vi "Heading.vi"(0 "X Array":dbl[](array[numeric]), 1 "Target X":dbl, 2 "Current X":dbl, 3 "Current Y":dbl, 4 "Target Y":dbl, 5 "Y Array":dbl[](array[numeric]), 7 "stop":bool) -> (6 "Current Heading":dbl, 8 "Desired Heading":dbl)   [LabVIEW 2012]
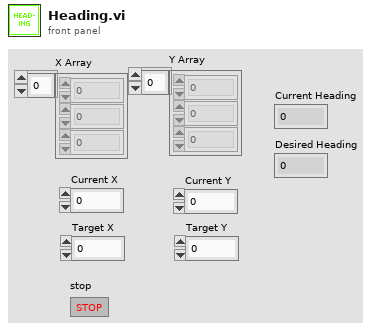
[diagram p1: front panel]
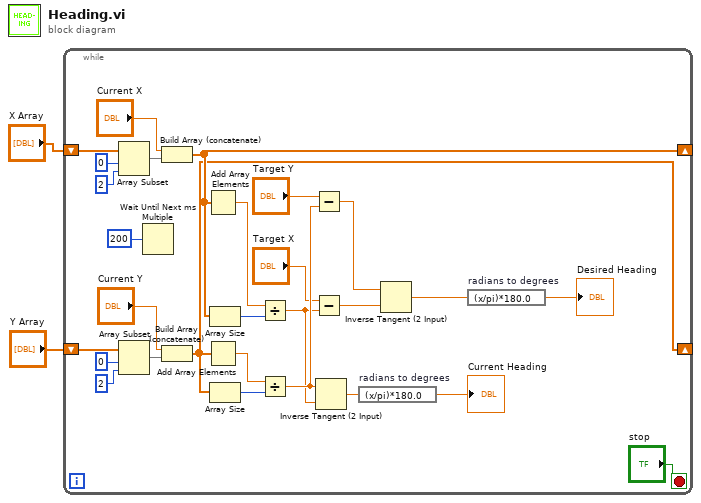
[diagram p0: block diagram]
diagram:
  n1 = while {
    shift-right: [w22] -> _
    shift-left: "X Array" -> [w30]
    shift-right: [w13] -> _
    shift-left: "Y Array" -> [w14]
    stop <- "stop" stop-if-true
    n2 = Array Subset(array=w30, index=0, length=2) -> (w27:dbl[])
    n3 = Array Subset(array=w14, index=0, length=2) -> (w18:dbl[])
    n4 = Wait Until Next ms Multiple(millisecond multiple=200) -> ()  [unwired: 1 out]
    n5 = Build Array (concatenate)("Current X", w27) -> (w22:dbl[])
    n6 = Build Array (concatenate)("Current Y", w18) -> (w13:dbl[])
    n7 = Add Array Elements(numeric array=w22) -> (sum=w23:dbl)
    n8 = Add Array Elements(numeric array=w13) -> (sum=w16:dbl)
    n9 = Array Size(array=w22) -> (size(s)=w21:i32)
    n10 = Array Size(array=w13) -> (size(s)=w15:i32)
    n11 = Divide(x=w23, y=w21) -> (x/y=w6:dbl)
    n12 = Divide(x=w16, y=w15) -> (x/y=w8:dbl)
    n13 = Subtract(x="Target Y", y=w8) -> (x-y=w10:dbl)
    n14 = Subtract(x="Target X", y=w6) -> (x-y=w5:dbl)
    n15 = Inverse Tangent (2 Input)(1:w6, 2:w8) -> (0:w12:dbl)
    n16 = expression code="(x/pi)*180.0" "radians to degrees"(w12) -> (→"Current Heading":dbl)
    n17 = Inverse Tangent (2 Input)(1:w5, 2:w10) -> (0:w4:dbl)
    n18 = expression code="(x/pi)*180.0" "radians to degrees"(w4) -> (→"Desired Heading":dbl)
  }
